vi "Build High Priority Async.vi"(6 "Group":i32, 7 "Virtual Memory Unit in":refnum<class "Virtual Memory Unit.lvclass">, 8 "error in (no error)":errorcluster, 10 "Starting Address":u16 format="%04x", 11 "Major Frame in":refnum<class "Major Frame.lvclass">) -> (0 "error out":errorcluster, 2 "Next Available Address":u16 format="%04x", 3 "Major Frame out":refnum<class "Major Frame.lvclass">, 5 "Virtual Memory Unit out":refnum<class "Virtual Memory Unit.lvclass">)   [LabVIEW 2020, in "BCI-1553 API.lvlib" / "Major Frame.lvclass"]
doc: "Creates a single High Priority Check, Execution, Configuration, and Data Field in memory. Requires 66 Registers for implementation."
uses:
  Major Frame.lvclass
  Dependencies/Virtual Memory Unit/Virtual Memory Unit.lvclass
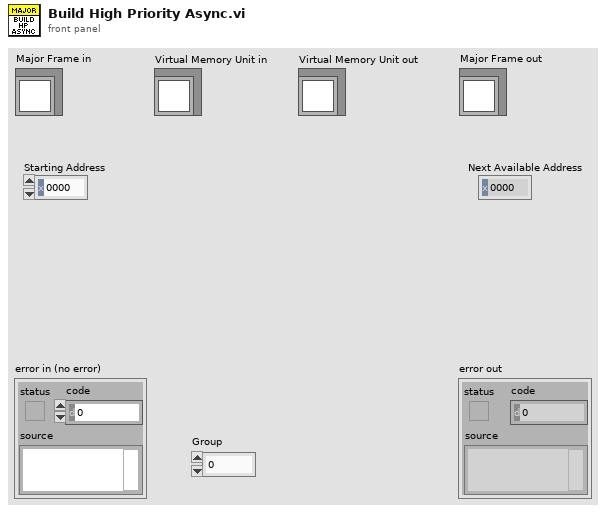
[diagram p1: front panel]
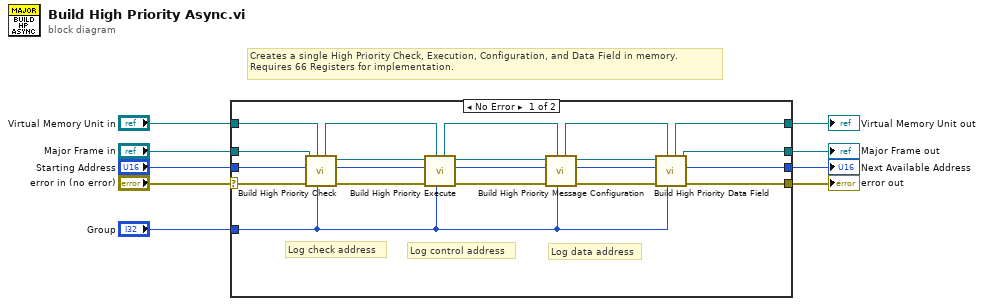
[diagram p0: block diagram]
diagram:
  # "Creates a single High Priority Check, Execution, Configuration, and Data Field in memory.\nRequires 66 Registers for implementation."
  n1 = case shown="No Error" "error in (no error)" {
    selector: "error in (no error)" -> [w25 w34]
    tunnel: [w24 w34] -> w8
    tunnel: [w26 w33] -> w7
    tunnel: "Major Frame in" -> [w27 w33]
    tunnel: "Virtual Memory Unit in" -> [w20 w32]
    tunnel: [w16 w32] -> w6
    tunnel: "Starting Address" -> [w15 w31]
    tunnel: [w11 w31] -> w4
    tunnel: "Group" -> [w10 _]
    frame No Error {
      # "Log data address"
      # "Log control address"
      # "Log check address"
      n2 = call "Build High Priority Check.vi"("Group"=w10, "Virtual Memory Unit in"=w20, "error in (no error)"=w25, "Starting Address"=w15, "Major Frame in"=w27) -> ("error out"=w23:errorcluster, "Next Available Address"=w14:u16, "Major Frame out"=w30:refnum<class "Major Frame.lvclass">, "Virtual Memory Unit out"=w19:refnum<class "Virtual Memory Unit.lvclass">)  [unwired: 3 in]
      n3 = call "Build High Priority Execute.vi"("Group"=w10, "Virtual Memory Unit in"=w19, "error in (no error)"=w23, "Starting Address"=w14, "Major Frame in"=w30) -> ("error out"=w22:errorcluster, "Next Available Address"=w13:u16, "Major Frame out"=w29:refnum<class "Major Frame.lvclass">, "Virtual Memory Unit out"=w18:refnum<class "Virtual Memory Unit.lvclass">)  [unwired: 3 in]
      n4 = call "Build High Priority Message Configuration.vi"("Group"=w10, "Virtual Memory Unit in"=w18, "error in (no error)"=w22, "Starting Address"=w13, "Major Frame in"=w29) -> ("error out"=w21:errorcluster, "Next Available Address"=w12:u16, "Major Frame out"=w28:refnum<class "Major Frame.lvclass">, "Virtual Memory Unit out"=w17:refnum<class "Virtual Memory Unit.lvclass">)  [unwired: 3 in]
      n5 = call "Build High Priority Data Field.vi"("Group"=w10, "Virtual Memory Unit in"=w17, "error in (no error)"=w21, "Starting Address"=w12, "Major Frame in"=w28) -> ("error out"=w24:errorcluster, "Next Available Address"=w11:u16, "Major Frame out"=w26:refnum<class "Major Frame.lvclass">, "Virtual Memory Unit out"=w16:refnum<class "Virtual Memory Unit.lvclass">)  [unwired: 3 in]
    }
    frame Error {
    }
  }
  "error out" <- w8
  "Major Frame out" <- w7
  "Virtual Memory Unit out" <- w6
  "Next Available Address" <- w4
